vi "RETR.vi"(8 "error in (no error)":errorcluster, 9 "Local FilePath":path, 10 "FileName":string, 11 "FTP in":refnum<class "FTP.lvclass">) -> (0 "error out":errorcluster, 3 "FTP out":refnum<class "FTP.lvclass">)   [LabVIEW 2020, in "FTP.lvlib" / "FTP.lvclass"]
uses:
  FTP.lvclass
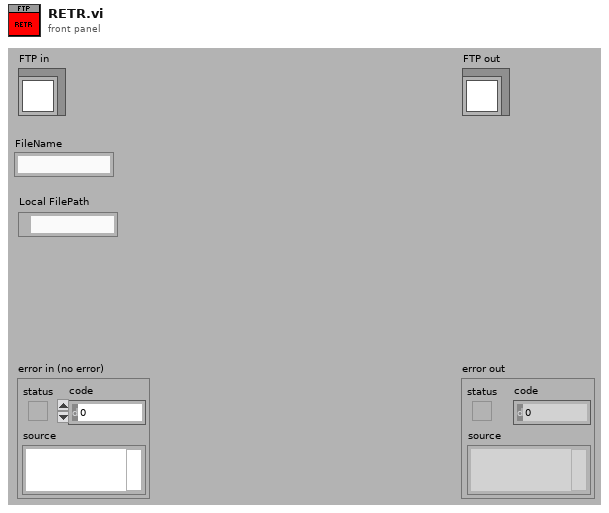
[diagram p1: front panel]
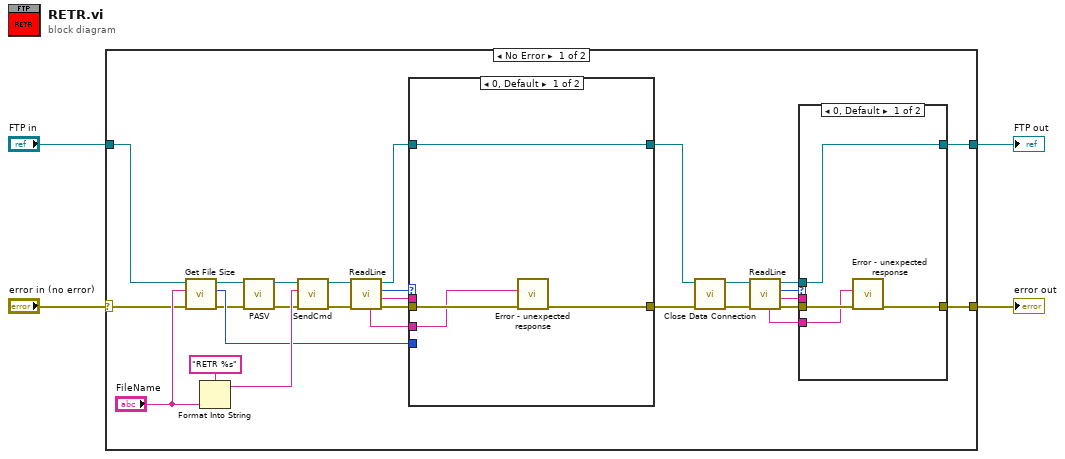
[diagram p0: block diagram]
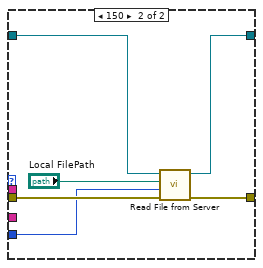
[diagram p2: hidden frame]
diagram:
  n1 = case shown="No Error" "error in (no error)" {
    selector: "error in (no error)" -> [w7 w50]
    tunnel: [w28 w50] -> w3
    tunnel: [w27 w49] -> w1
    tunnel: "FTP in" -> [w8 w49]
    frame No Error {
      n2 = call "Get File Size.vi"("error in (no error)"=w7, "Remote FileName"="FileName", "FTP in"=w8) -> ("error out"=w12:errorcluster, "FileSize"=w13:i64, "FTP out"=w11:refnum<class "FTP.lvclass">)  [unwired: 6 in]
      n3 = Format Into String(format string="RETR %s" ("cmd"), "FileName") -> (resulting string=w25:string)  [unwired: 2 in, 1 out]
      n4 = call "PASV.vi"("error in (no error)"=w12, "FTP in"=w11) -> ("error out"=w9:errorcluster, "FTP out"=w10:refnum<class "FTP.lvclass">)  [unwired: 8 in]
      n5 = call "SendCmd.vi"("error in (no error)"=w9, "cmd"=w25, "FTP in"=w10) -> ("error out"=w31:errorcluster, "FTP out"=w32:refnum<class "FTP.lvclass">)  [unwired: 7 in]
      n6 = call "ReadLine.vi"("error in (no error)"=w31, "FTP in"=w32) -> ("error out"=w30:errorcluster, "Line"=w15:string, "code"=w16:i32, "FTP out"=w29:refnum<class "FTP.lvclass">, "Full Line"=w6:string)  [unwired: 5 in]
      n7 = case shown="0, Default" w16 {
        tunnel: w30 -> [w35 w42]
        tunnel: w29 -> [w36 w41]
        tunnel: [w34 w38] -> w18
        tunnel: [w36 w40] -> w17
        tunnel: w15 -> [_ _]
        tunnel: w13 -> [_ w39]
        tunnel: w6 -> [w33 _]
        frame 0, Default {
          n8 = call "Error - unexpected response.vi"("error in (no error)"=w35, "Full Response"=w33) -> ("error out"=w34:errorcluster)  [unwired: 9 in]
        }
        frame 150 {
          n9 = call "Read File from Server.vi"("error in (no error)"=w42, "FileSize"=w39, "Local FilePath"="Local FilePath", "FTP in"=w41) -> ("error out"=w38:errorcluster, "FTP out"=w40:refnum<class "FTP.lvclass">)  [unwired: 6 in]
        }
      }
      n10 = call "Close Data Connection.vi"("error in (no error)"=w18, "FTP in"=w17) -> ("error out"=w24:errorcluster, "FTP out"=w23:refnum<class "FTP.lvclass">)  [unwired: 8 in]
      n11 = call "ReadLine.vi"("error in (no error)"=w24, "FTP in"=w23) -> ("error out"=w22:errorcluster, "Line"=w19:string, "code"=w21:i32, "FTP out"=w20:refnum<class "FTP.lvclass">, "Full Line"=w5:string)  [unwired: 5 in]
      n12 = case shown="0, Default" w21 {
        tunnel: w22 -> [w45 w47]
        tunnel: [w44 w47] -> w28
        tunnel: w20 -> [w46 w48]
        tunnel: [w46 w48] -> w27
        tunnel: w19 -> [_ _]
        tunnel: w5 -> [w43 _]
        frame 0, Default {
          n13 = call "Error - unexpected response.vi"("error in (no error)"=w45, "Full Response"=w43) -> ("error out"=w44:errorcluster)  [unwired: 9 in]
        }
        frame 226 {
        }
      }
    }
    frame Error {
    }
  }
  "error out" <- w3
  "FTP out" <- w1
